vi "test_FXP Signed Value Conversion_I8.vi"(8 "error in (no error)":errorcluster, 11 "TestCase in":refnum<class "FPGA Register IO Tests.lvclass">) -> (0 "error out":errorcluster, 3 "TestCase out":refnum<class "FPGA Register IO Tests.lvclass">)   [LabVIEW 2018, in "FPGA Register IO Tests.lvclass"]
uses:
  FPGA Register IO Tests.lvclass
  APIs/FPGA Register IO/TypeDefs/FXP Configuration.ctl
  <vilib>/fxp/LVFixedPointRepBitsTypeDef.ctl
  <vilib>/fxp/LVFixedPointRepRangeTypeDef.ctl
  <vilib>/addons/_JKI Toolkits/VI Tester/TestCase.llb/TestCase.lvclass
  APIs/FPGA Register IO/FPGA Register IO.lvlib
  <vilib>/Utility/Data Type/NI_Data Type.lvlib
  C:/Program Files (x86)/National Instruments/LabVIEW 2018/vi.lib/addons/_JKI Toolkits/VI Tester/TestCase.llb/TestCase.lvclass
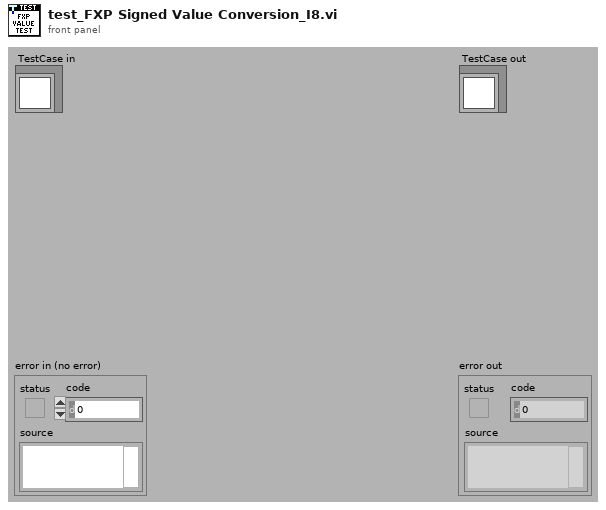
[diagram p1: front panel]
types:
  T1 = typedef "FPGA Register IO.lvlib/FXP Configuration.ctl" = cluster{"FXP Representation":T2, "FXP Range":T3}
  T2 = typedef "LVFixedPointRepBitsTypeDef.ctl" = cluster{"Signed":bool, "Word Length":u32, "Integer Word Length":i32}
  T3 = typedef "LVFixedPointRepRangeTypeDef.ctl" = cluster{"Range Min":dbl, "Range Max":dbl, "Delta":dbl}
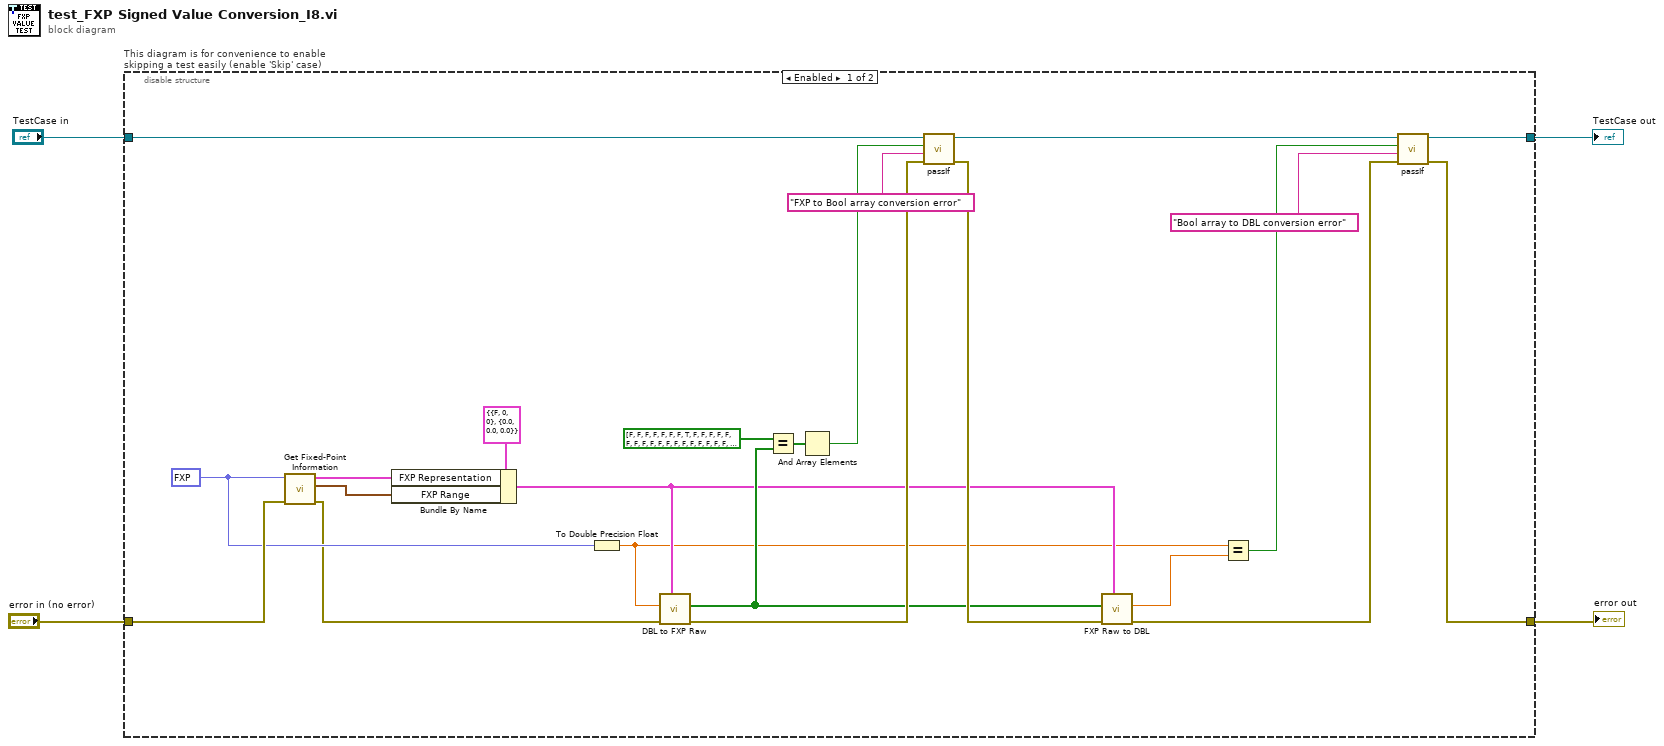
[diagram p0: block diagram]
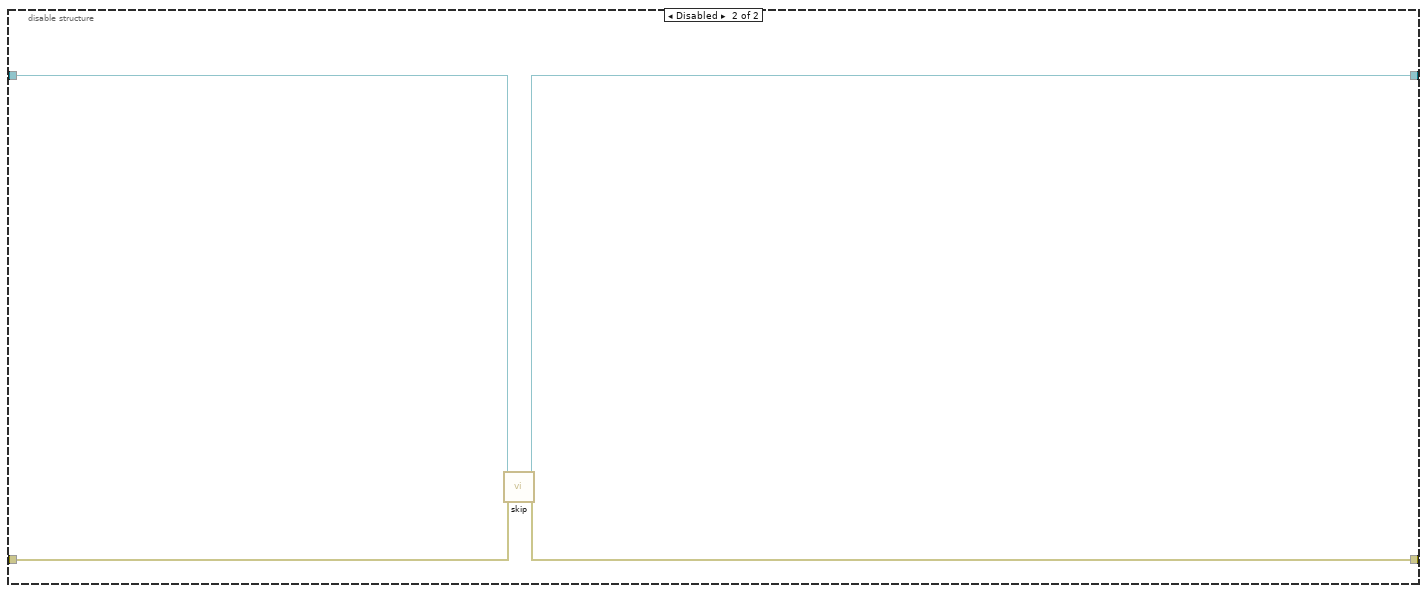
[diagram p2: hidden frame]
diagram:
  n1 = disable-structure "This diagram is for convenience to enable skipping a test easily (enable 'Skip' case)" shown="Enabled" {
    disable-tunnel: "TestCase in" -> [w20 w31]
    disable-tunnel: [w7 w29] -> w1
    disable-tunnel: [w8 w30] -> w3
    disable-tunnel: "error in (no error)" -> [w24 w28]
    frame Enabled {
      w23 = fxp<+/-,8,8> -128.0
      n2 = call <vilib>:"Get Fixed-Point Information.vi"("error in (no error)"=w24, "Variant"=w23) -> ("error out"=w22:errorcluster, "FXP Range"=w25:T3, "FXP Representation"=w26:T2)  [unwired: 6 in, 1 out]
      n3 = Bundle By Name(cluster=T1 {"FXP Representation"={"Signed"=FALSE, "Word Length"=0, "Integer Word Length"=0}, "FXP Range"={"Range Min"=0.0, "Range Max"=0.0, "Delta"=0.0}} ("FXP Configuration"), "FXP Representation"=w26, "FXP Range"=w25) -> (w14:T1)
      n4 = To Double Precision Float(number=w23) -> (double precision float=w12:dbl)
      n5 = call "DBL to FXP Raw.vi"("FXP Configuration"=w14, "error in (no error)"=w22, "DBL Value"=w12) -> ("error out"=w19:errorcluster, "Bool Data"=w15:bool[])  [unwired: 7 in]
      n6 = Equal?(x=bool[] [FALSE, FALSE, FALSE, FALSE, FALSE, FALSE, FALSE, TRUE, FALSE, FALSE, FALSE, FALSE, FALSE, FALSE, FALSE, FALSE, FALSE, FALSE, FALSE, FALSE, FALSE, FALSE, FALSE, FALSE, FALSE, FALSE, FALSE, FALSE, FALSE, FALSE, FALSE, FALSE, FALSE, FALSE, FALSE, FALSE, FALSE, FALSE, FALSE, FALSE, FALSE, FALSE, FALSE, FALSE, FALSE, FALSE, FALSE, FALSE, FALSE, FALSE, FALSE, FALSE, FALSE, FALSE, FALSE, FALSE, FALSE, FALSE, FALSE, FALSE, FALSE, FALSE, FALSE, FALSE] ("Bool Data"), y=w15) -> (x = y?=w21:bool[])
      n7 = And Array Elements(Boolean array=w21) -> (logical AND=w18:bool)
      n8 = call-dynamic "passIf.vi"("error in (no error)"=w19, "message (\"\")"="FXP to Bool array conversion error" ("message (\"\")"), "pass"=w18, "TestCase in"=w20) -> ("error out"=w17:errorcluster, "TestCase out"=w11:refnum<class "FPGA Register IO Tests.lvclass">)  [unwired: 6 in]
      n9 = call "FXP Raw to DBL.vi"("FXP Configuration"=w14, "error in (no error)"=w17, "Bool Data"=w15) -> ("error out"=w9:errorcluster, "DBL Value"=w13:dbl)  [unwired: 7 in]
      n10 = Equal?(x=w12, y=w13) -> (x = y?=w10:bool)
      n11 = call-dynamic "passIf.vi"("error in (no error)"=w9, "message (\"\")"="Bool array to DBL conversion error" ("message (\"\")"), "pass"=w10, "TestCase in"=w11) -> ("error out"=w8:errorcluster, "TestCase out"=w7:refnum<class "FPGA Register IO Tests.lvclass">)  [unwired: 6 in]
    }
    frame Disabled {
      # "skip test result while test is under development"
      n12 = call <vilib>:"skip.vi"("error in (no error)"=w28, "TestCase in"=w31) -> ("error out"=w30:errorcluster, "TestCase out"=w29:refnum<class "FPGA Register IO Tests.lvclass">)  [unwired: 8 in]
    }
  }
  "error out" <- w3
  "TestCase out" <- w1
